vi "signalgen_2.vi"() -> ()   [LabVIEW 2013]
uses:
  <vilib>/Analysis/1siggen.llb/Ramp Pattern by Samples.vi
  <vilib>/Analysis/NI_AALBase.lvlib
panel:
  out "error out":errorcluster
  out "VISA resource name out":refnum<visa-resource-name>
  in  "VISA resource name 3":refnum<visa-resource-name>
  in  "error in (no error) 3":errorcluster
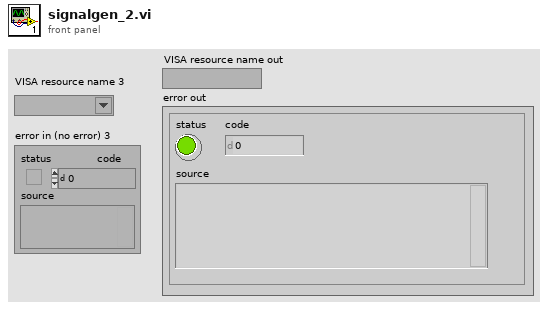
[diagram p1: front panel]
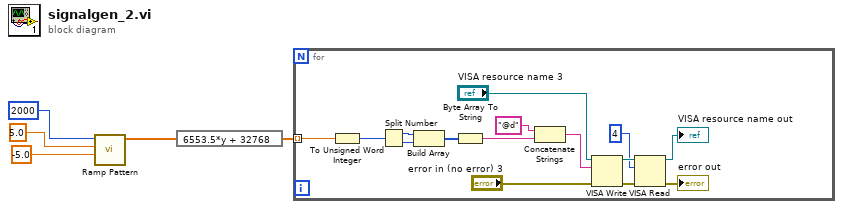
[diagram p0: block diagram]
diagram:
  n1 = call-poly <vilib>:"Ramp Pattern.vi"("start"=-5.0, "end"=5.0, "samples"=2000) -> ("Ramp Pattern"=w1:dbl[])  [unwired: 7 in, 1 out]
  n2 = expression code="6553.5*y + 32768"(w1) -> (w3:dbl[])
  n3 = for {
    tunnel: w3 -> [w6] mode=indexing
    n4 = To Unsigned Word Integer(number=w6) -> (unsigned 16bit integer=w19:u16)
    n5 = Split Number(x=w19) -> (hi(x)=w16:u8, lo(x)=w17:u8)
    n6 = Build Array(w16, w17) -> (w20:u8[])
    n7 = Byte Array To String(unsigned byte array=w20) -> (string=w18:string)
    n8 = Concatenate Strings("@d" ("write buffer"), w18) -> (w10:string)
    n9 = VISA Write(VISA resource name="VISA resource name 3", write buffer=w10, error in (no error)="error in (no error) 3") -> (VISA resource name out=w12:refnum<visa-resource-name>, error out=w13:errorcluster)  [unwired: 1 out]
    n10 = VISA Read(VISA resource name=w12, byte count=u32 4, error in (no error)=w13) -> (VISA resource name out=→"VISA resource name out":refnum<visa-resource-name>, error out=→"error out":errorcluster)  [unwired: 2 out]
  }
